vi "Matlab Param Array to String.vi"(8 "error in (no error)":errorcluster, 10 "Name":string, 11 "Matlab Param Array":cluster{"Name":string, "Data":variant}[](array[cluster])) -> (0 "error out":errorcluster, 3 "data":string)   [LabVIEW 2014, in "Matlab API.lvlib"]
uses:
  Matlab API.lvlib
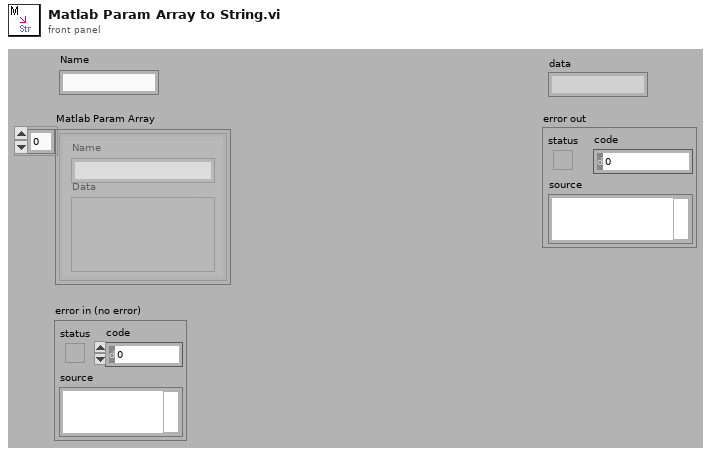
[diagram p1: front panel]
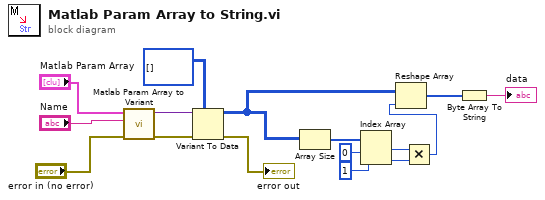
[diagram p0: block diagram]
diagram:
  n1 = call "Matlab Param Array to Variant.vi"("error in (no error)"="error in (no error)", "Name"="Name", "Variables"="Matlab Param Array") -> ("error out"=w15:errorcluster, "Data"=w16:variant)  [unwired: 7 out]
  n2 = Variant To Data(error in=w15, type=u8[][] [], Variant=w16) -> (data=w9:u8[][], error out=→"error out":errorcluster)
  n3 = Array Size(array=w9) -> (size(s)=w6:i32[])
  n4 = Index Array(array=w6, index #1=0 ("index"), index #2=1 ("index")) -> (element #1=w4:i32, element #2=w5:i32)
  n5 = Multiply(x=w4, y=w5) -> (x*y=w3:i32)
  n6 = Reshape Array(w9, w3) -> (w2:u8[])
  n7 = Byte Array To String(unsigned byte array=w2) -> (string=→"data":string)
